vi "Get Hide Lines.vi"(9 "Recording Cluster":T1) -> (2 "Num of hidden Lines":u32)   [LabVIEW 2017, in "Digital_Group.xnode"]
uses:
  <vilib>/express/express signal manip/DigitalDataGroupingXNode/Digital_Group.xnode
  <vilib>/express/express signal manip/DigitalDataGroupingXNode/DigitalGroup_Recording Cluster.ctl
panel:
  # "When some of the buses are closed, the Lines under the closed buses will be hidden.\nThis VI get the whole hidden Lines.\nThe reason for this VI is for setting Digital Waveform Graph."
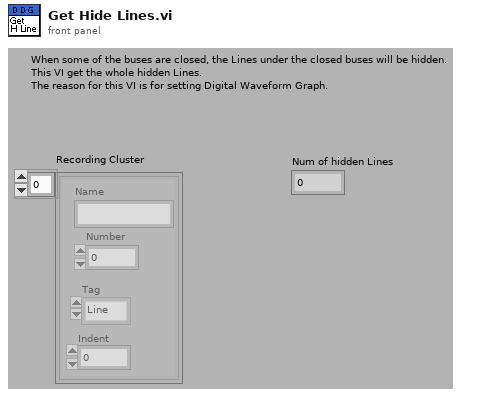
[diagram p1: front panel]
types:
  T1 = typedef "DigitalGroup_Recording Cluster.ctl" = cluster{"Name":string, "Number":u32, "Indent":u32, "Tag":enum16{"Line", "Opened Bus", "Closed Bus"}}[]
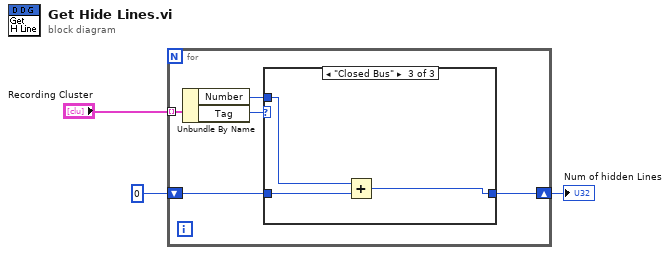
[diagram p0: block diagram]
diagram:
  n1 = for {
    tunnel: "Recording Cluster" -> [w8] mode=indexing
    shift-right: [w5] -> w1
    shift-left: u32 0 -> [w6]
    n2 = Unbundle By Name(w8) -> ("Number"=w4:u32, "Tag"=w7:enum16{"Line", "Opened Bus", "Closed Bus"})
    n3 = case shown="\"Closed Bus\"" w7 {
      tunnel: w6 -> [w9 w10 w12]
      tunnel: [w9 w10 w11] -> w5
      tunnel: w4 -> [_ _ w13]
      frame "Line", Default {
      }
      frame "Opened Bus" {
      }
      frame "Closed Bus" {
        n4 = Add(x=w13, y=w12) -> (x+y=w11:u32)
      }
    }
  }
  "Num of hidden Lines" <- w1
